vi "getValid.vi"(8 "error in (no error)":errorcluster, 11 "ReaderStatus in":refnum<class "IReaderStatus.lvclass">) -> (0 "error out":errorcluster, 2 "isValid?":bool, 3 "ReaderStatus out":refnum<class "IReaderStatus.lvclass">)   [LabVIEW 2022 SP3, in "openDAQ.lvlib" / "IBaseObject.lvlib" / "IReaderStatus.lvlib" / "IReaderStatus.lvclass"]
uses:
  <instrlib>/openDAQ/Public/Classes/IReaderStatus/IReaderStatus.lvclass
  C:/Program Files (x86)/National Instruments/LabVIEW 2022/instr.lib/openDAQ/Public/Classes/IBaseObject/IBaseObject.lvclass
  <instrlib>/openDAQ/Public/Classes/IBaseObject/IBaseObject.lvclass/IBaseObject.ctl
  <instrlib>/openDAQ/Public/Classes/IBaseObject/Accessor/Read reference.vi
  <instrlib>/openDAQ/Public/Classes/IReaderStatus/IReaderStatus.lvclass/IReaderStatus.ctl
  <instrlib>/openDAQ/Binaries/Windows/x86/copendaq32.dll
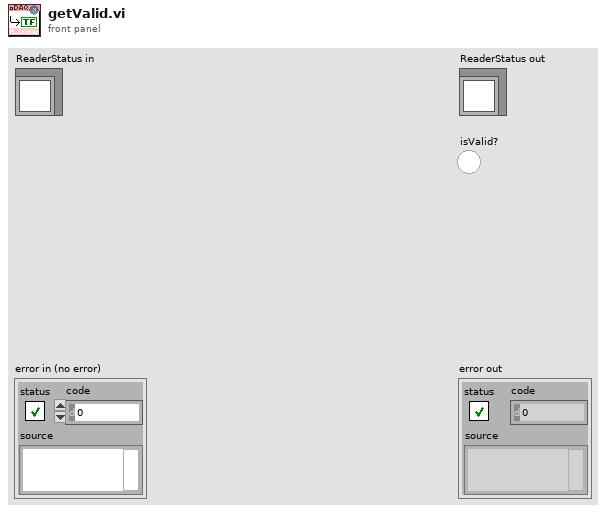
[diagram p1: front panel]
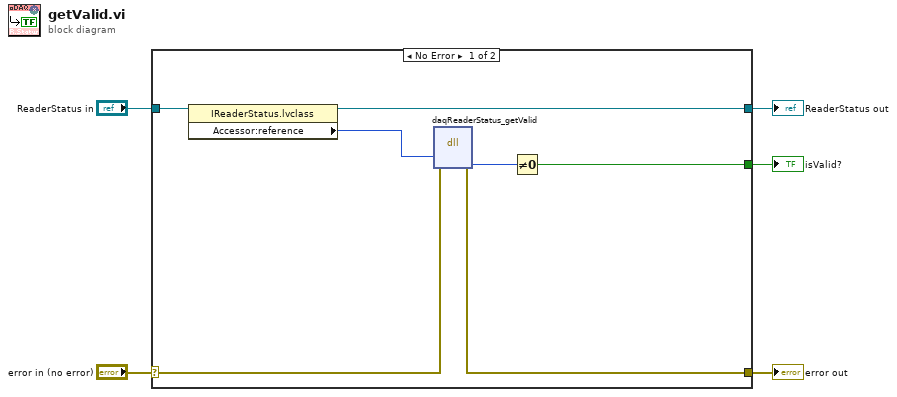
[diagram p0: block diagram]
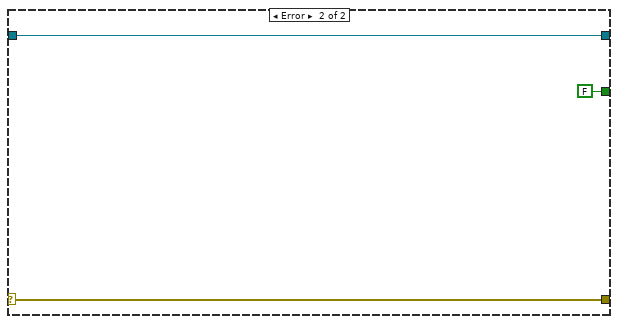
[diagram p2: hidden frame]
diagram:
  n1 = case shown="No Error" "error in (no error)" {
    selector: "error in (no error)" -> [w6 w15]
    tunnel: [w7 w15] -> w4
    tunnel: [w11 w14] -> w2
    tunnel: "ReaderStatus in" -> [w12 w14]
    tunnel: [w8 FALSE] -> w1
    frame No Error {
      n2 = property class="IReaderStatus.lvclass"(reference=w12) -> (reference out=w11:refnum<class "IReaderStatus.lvclass">, "Accessor:reference"=w10:i64)  [unwired: 1 in, 1 out]
      n3 = dll-call lib="C:/Program Files (x86)/National Instruments/LabVIEW 2022/instr.lib/openDAQ/Binaries/Windows/x86/copendaq*.*" fn="daqReaderStatus_getValid"(error in=w6, "readerStatus"=w10) -> (error out=w7:errorcluster, "valid"=w9:i64)  [unwired: 5 in, 1 out]
      n4 = Not Equal To 0?(x=w9) -> (x != 0?=w8:bool)
    }
    frame Error {
    }
  }
  "error out" <- w4
  "ReaderStatus out" <- w2
  "isValid?" <- w1
